vi "Dashboard Main.vi"() -> ()   [LabVIEW 2011]
uses:
  2013 Robot Code 11-1-12/Dashboard Datatype.ctl
  <vilib>/Rock Robotics/WPI/DriverStation/WPI_DriverStationDigitalData.ctl
panel:
  in  "Viewer":enum32{"Camera Image", "Kinect Skeleton", "IO"}(tab)
  in  "Video Left Enable":bool=TRUE
  out "Default Camera Left":T1(plugin-control)
  out "Camera Right":T1(plugin-control)
  in  "Video Right Enable":bool=TRUE
  out "Auton Name 1":string
  out "Auton Name 2":string
  out "Auton Name 3":string
  out "Auton Name 4":string
  out "Auton Name 5":string
  out "Auton Name 6":string
  out "Buttons 1":cluster{"1":bool, "2":bool, "3":bool}
  out "Kinect 1":cluster{"X":dbl, "Y":dbl, "Z":dbl} {"X" scale=1.0..-1.0; "Y" scale=1.0..-1.0; "Z" scale=1.0..-1.0}
  out "Buttons 2":cluster{"1":bool, "2":bool, "3":bool}
  out "Kinect 2":cluster{"X":dbl, "Y":dbl, "Z":dbl} {"X" scale=1.0..-1.0; "Y" scale=1.0..-1.0; "Z" scale=1.0..-1.0}
  out "Version":string
  out "Skeleton Picture":picture
  out "Players":i8
  out "PWM":cluster{u8, u8}[](array[slide])=[{0, 157}, {0, 157}, {0, 157}, {0, 157}, {0, 157}, {0, 157}, {0, 157}, {0, 157}, {0, 157}, {0, 169}] scale=1.0..255.0
  out "GPIO Output Enable":bool[](array[boolean])
  out "GPIO State":bool[](array[boolean])
  out "Relay":cluster{"Forward":bool[], "Reverse":bool[]}
  out "Solenoid Output":bool[](array[boolean])
  out "Robot IP Address":string
  out "8 -- Battery":sgl(graph)
  out "Analog Input":sgl[](array[slide]) scale=0.0..5.0
  out "Dashboard Datatype Warning":string="Warning: The Dashboard Datatype used by the robot project and this dashboard do not match.\nSee diagram for more details."
  out "Image Error Message":string="Timeout in Camera Communications"
  # "Digital #1"
  # "1"
  # "10"
  # "1"
  # "14"
  # "1"
  # "8"
  # "Solenoid #1"
  # "1"
  # "8"
  # "Communications"
  # "Analog #1"
  # "1"
  # "7"
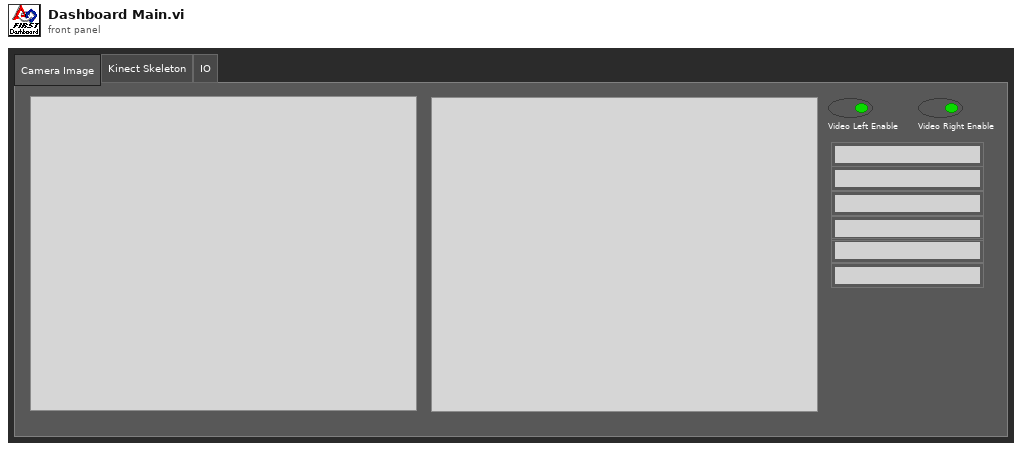
[diagram p1: front panel]
types:
  T1 = typedef "IMAQ Image.ctl" = refnum<image>
  T2 = typedef "Dashboard Datatype.ctl" = cluster{cluster{"AnalogModule[0]":cluster{"Channel[0]":sgl, "Channel[1]":sgl, "Channel[2]":sgl, "Channel[3]":sgl, "Channel[4]":sgl, "Channel[5]":sgl, "Channel[6]":sgl, "Channel[7]":sgl}, "AnalogModule[1]":cluster{"Channel[0]":sgl, "Channel[1]":sgl, "Channel[2]":sgl, "Channel[3]":sgl, "Channel[4]":sgl, "Channel[5]":sgl, "Channel[6]":sgl, "Channel[7]":sgl}}, cluster{"DigitalModule[0]":T3, "DigitalModule[1]":T3}, "Solenoid":u8, "Auton Files":string[]}
  T3 = typedef "WPI_DriverStationDigitalData.ctl" = cluster{"Relay Fwd":u8, "Relay Rev":u8, "GPIO":u16, "GPIO_OE":u16, "PWM":cluster{"PWM[0]":u8, "PWM[1]":u8, "PWM[2]":u8, "PWM[3]":u8, "PWM[4]":u8, "PWM[5]":u8, "PWM[6]":u8, "PWM[7]":u8, "PWM[8]":u8, "PWM[9]":u8}}
  T4 = typedef "Image Type" = u32
  T5 = cluster{"Competition mode":bool, "Robot Link":bool, "Autonomous":bool, "Enabled":bool, "E-Stop":bool}
  T6 = cluster{"AnalogModule[0]":cluster{"Channel[0]":sgl, "Channel[1]":sgl, "Channel[2]":sgl, "Channel[3]":sgl, "Channel[4]":sgl, "Channel[5]":sgl, "Channel[6]":sgl, "Channel[7]":sgl}, "AnalogModule[1]":cluster{"Channel[0]":sgl, "Channel[1]":sgl, "Channel[2]":sgl, "Channel[3]":sgl, "Channel[4]":sgl, "Channel[5]":sgl, "Channel[6]":sgl, "Channel[7]":sgl}}
  T7 = cluster{"DigitalModule[0]":T3, "DigitalModule[1]":T3}
  T8 = cluster{"Channel[0]":sgl, "Channel[1]":sgl, "Channel[2]":sgl, "Channel[3]":sgl, "Channel[4]":sgl, "Channel[5]":sgl, "Channel[6]":sgl, "Channel[7]":sgl}[]
  T9 = cluster{"Channel[0]":sgl, "Channel[1]":sgl, "Channel[2]":sgl, "Channel[3]":sgl, "Channel[4]":sgl, "Channel[5]":sgl, "Channel[6]":sgl, "Channel[7]":sgl}
  T10 = typedef "LVRectTypeDef.ctl" = cluster{"left":i16, "top":i16, "right":i16, "bottom":i16}
  T11 = typedef "SkeletonTrackState.ctl" = enum32{"NotTracked", "PositionOnly", "Tracked"}
  T12 = cluster{"TrackingState":u8[], "Position":cluster{"x":sgl, "y":sgl, "z":sgl}, cluster{"x":sgl, "y":sgl, "z":sgl, sgl}[], "TrackState":T11}
  T13 = cluster{cluster{"ScaledToPercentRange":dbl, "ScaledToPercentRange":dbl, "ScaledToPercentRange":dbl}, cluster{bool, bool, bool}}[]
  T14 = typedef "LVBoundsTypeDef.ctl" = cluster{"Width":u32, "Height":u32}
  T15 = cluster{cluster{"ScaledToPercentRange":dbl, "ScaledToPercentRange":dbl, "ScaledToPercentRange":dbl}, cluster{bool, bool, bool}}
  T16 = cluster{"ScaledToPercentRange":dbl, "ScaledToPercentRange":dbl, "ScaledToPercentRange":dbl}
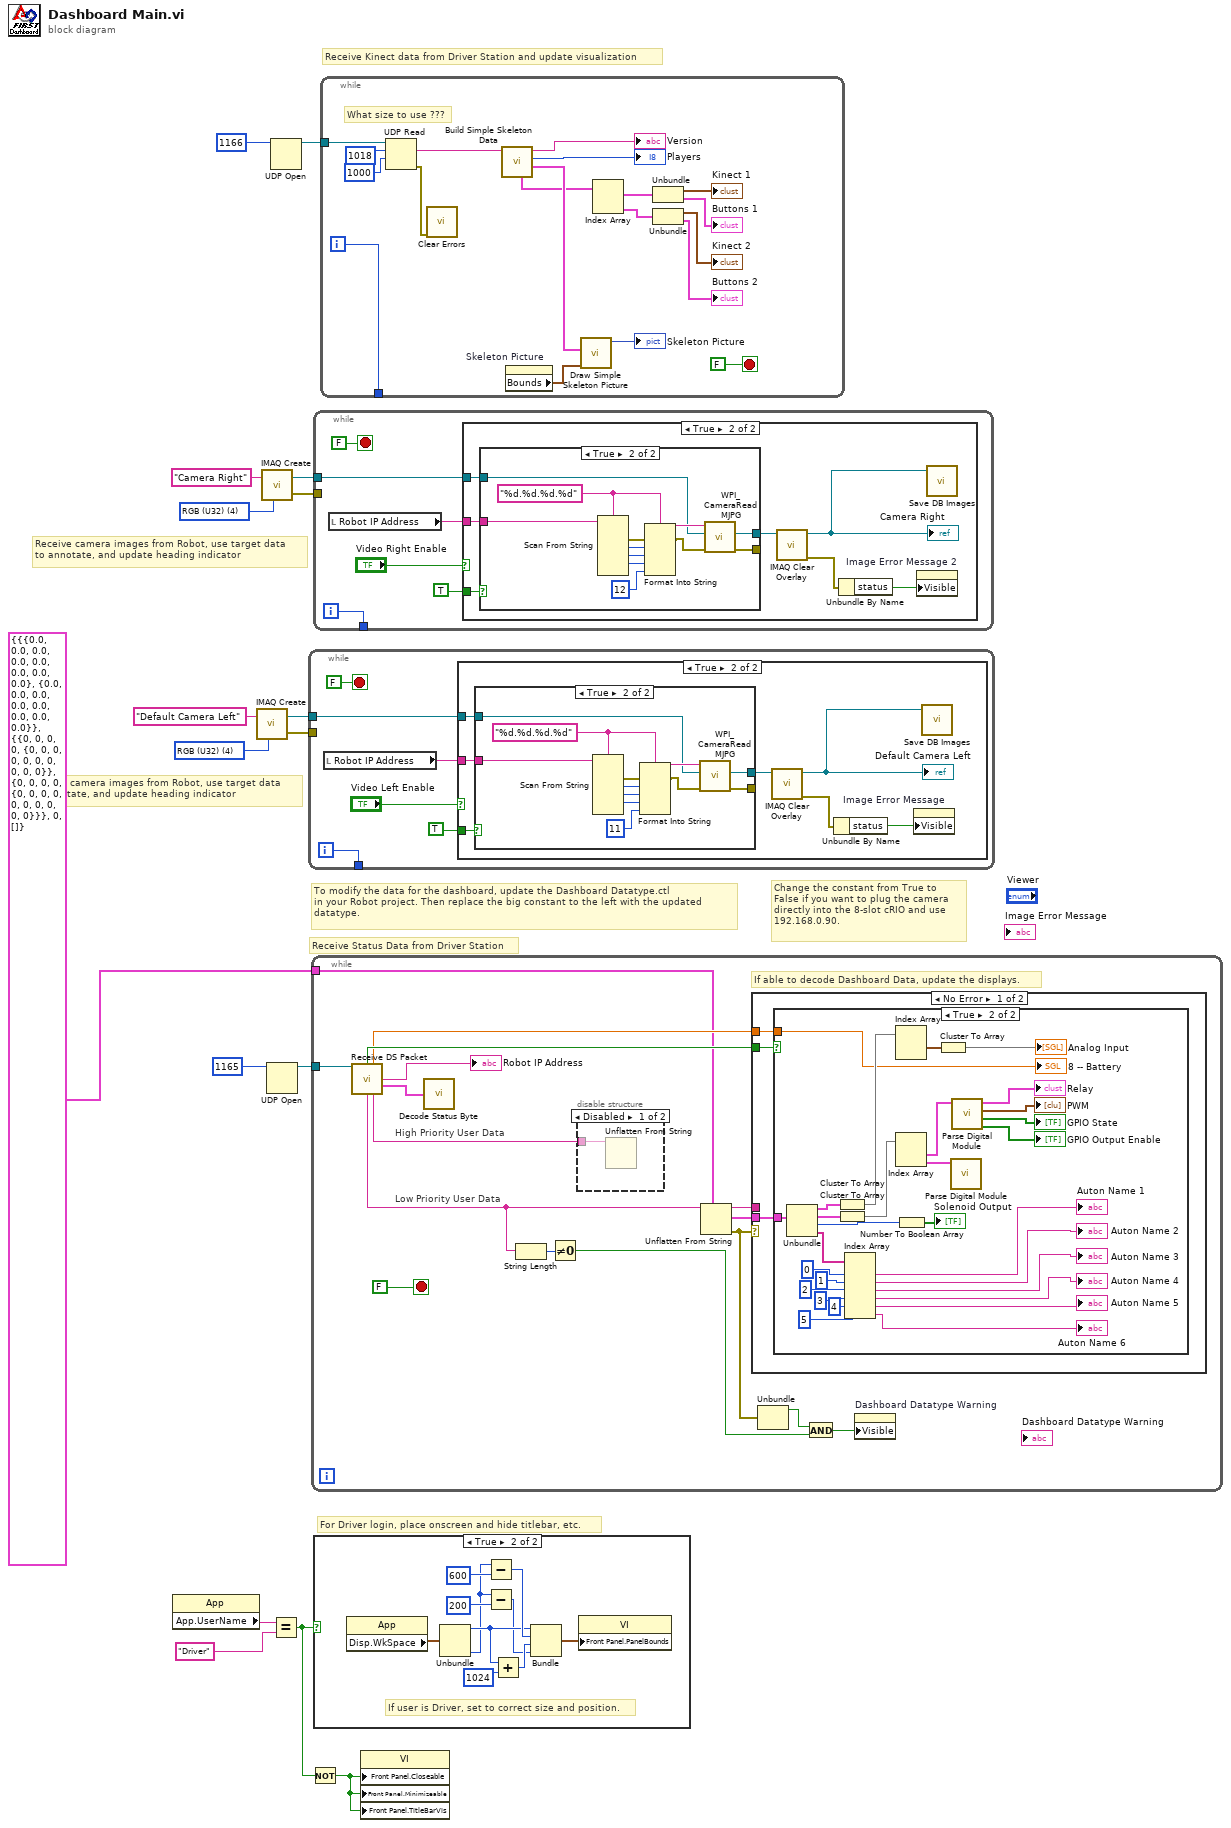
[diagram p0: block diagram]
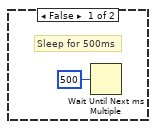
[diagram p2: hidden frame]
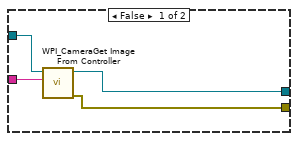
[diagram p3: hidden frame]
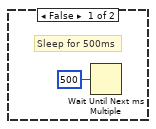
[diagram p8: hidden frame]
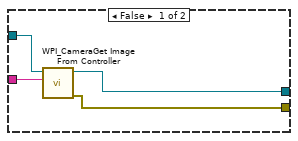
[diagram p9: hidden frame]
diagram:
  w5 = T4 4 items=["Grayscale (U8)", "Grayscale (I16)", "Grayscale (SGL)", "Complex (CSG)", "RGB (U32)", "HSL (U32)", "RGB (U64)"] ("Image Type")
  w15 = T4 4 items=["Grayscale (U8)", "Grayscale (I16)", "Grayscale (SGL)", "Complex (CSG)", "RGB (U32)", "HSL (U32)", "RGB (U64)"] ("Image Type")
  # "Receive camera images from Robot, use target data\nto annotate, and update heading indicator"
  # "Change the constant from True to\nFalse if you want to plug the camera\ndirectly into the 8-slot cRIO and use\n192.168.0.90."
  # "Receive Kinect data from Driver Station and update visualization"
  # "For Driver login, place onscreen and hide titlebar, etc."
  # "To modify the data for the dashboard, update the Dashboard Datatype.ctl\nin your Robot project. Then replace the big constant to the left with the updated\ndatatype."
  # "Receive Status Data from Driver Station"
  # "Receive camera images from Robot, use target data\nto annotate, and update heading indicator"
  n1 = property class="App"() -> ("App.UserName"=w10:string)  [unwired: 2 in, 2 out]
  n2 = call "IMAQ Create"("Image Name"="Default Camera Left", "Image Type"=w15) -> ("New Image"=w13:T1, "error out"=w12:errorcluster)  [unwired: 2 in, 1 out]
  n3 = call "IMAQ Create"("Image Name"="Camera Right", "Image Type"=w5) -> ("New Image"=w3:T1, "error out"=w2:errorcluster)  [unwired: 2 in, 1 out]
  n4 = UDP Open(11:u16 1165 ("port")) -> (port=w16:refnum<k16>)  [unwired: 2 in, 4 out]
  n5 = UDP Open(11:u16 1166 ("port")) -> (port=w6:refnum<k16>)  [unwired: 2 in, 4 out]
  n6 = Equal?(x=w10, y="Driver") -> (x = y?=w9:bool)
  n7 = while {
    tunnel: w13 -> [w21]
    tunnel: w12 -> [_]
    tunnel: [w18] -> _
    i -> [w18]
    stop <- FALSE stop-if-true
    n8 = local read "Robot IP Address"() -> (w22:string)
    n9 = case shown="True" "Video Left Enable" {
      tunnel: w22 -> [_ w31]
      tunnel: w21 -> [_ w30]
      tunnel: TRUE -> [_ w25]
      frame False {
        # "Sleep for 500ms"
        n10 = Wait Until Next ms Multiple(millisecond multiple=u32 500) -> ()  [unwired: 1 out]
      }
      frame True {
        n11 = case shown="True" w25 {
          tunnel: w30 -> [w34 w41]
          tunnel: [w32 w39] -> _
          tunnel: [w33 w40] -> w27
          tunnel: w31 -> [w35 w44]
          frame False {
            n12 = call <vilib>:"WPI_CameraGet Image From Controller.vi"("Controller Address"=w35, "Image"=w34) -> ("error out"=w32:errorcluster, "Image Out"=w33:T1)  [unwired: 2 in, 6 out]
          }
          frame True {
            w36 = "%d.%d.%d.%d" ("format string")
            n13 = Scan From String(format string=w36, input string=w44) -> (error out=w43:errorcluster, output 1=w45:i32, output 2=w46:i32, output 3=w47:i32)  [unwired: 2 in, 7 out]
            n14 = Format Into String(format string=w36, error in=w43, w45, w46, w47, 11 ("IP Suffix:")) -> (resulting string=w42:string, error out=w38:errorcluster)  [unwired: 1 in]
            n15 = call <vilib>:"WPI_CameraRead MJPG.vi"("error in"=w38, "Image"=w41, "address"=w42) -> ("error out"=w39:errorcluster, "Image Out"=w40:T1)  [unwired: 7 in]
          }
        }
        n16 = call "IMAQ Clear Overlay"("Image"=w27) -> ("error out"=w28:errorcluster, "Image Out"=w26:T1)  [unwired: 2 in, 7 out]
        "Default Camera Left" <- w26
        n17 = Unbundle By Name(w28) -> ("status"=w29:bool)
        n18 = property on="Image Error Message" class="Str"("Visible"=w29) -> ()  [unwired: 2 in, 2 out]
        n19 = call "Save DB Images.vi"("Image"=w26) -> ()  [unwired: 2 in, 1 out]
      }
    }
  }
  n20 = Not(x=w9) -> (.not. x?=w8:bool)
  n21 = while {
    tunnel: w16 -> [w61]
    tunnel: T2 {{"AnalogModule[0]"={"Channel[0]"=0.0, "Channel[1]"=0.0, "Channel[2]"=0.0, "Channel[3]"=0.0, "Channel[4]"=0.0, "Channel[5]"=0.0, "Channel[6]"=0.0, "Channel[7]"=0.0}, "AnalogModule[1]"={"Channel[0]"=0.0, "Channel[1]"=0.0, "Channel[2]"=0.0, "Channel[3]"=0.0, "Channel[4]"=0.0, "Channel[5]"=0.0, "Channel[6]"=0.0, "Channel[7]"=0.0}}, {"DigitalModule[0]"={"Relay Fwd"=0, "Relay Rev"=0, "GPIO"=0, "GPIO_OE"=0, "PWM"={"PWM[0]"=0, "PWM[1]"=0, "PWM[2]"=0, "PWM[3]"=0, "PWM[4]"=0, "PWM[5]"=0, "PWM[6]"=0, "PWM[7]"=0, "PWM[8]"=0, "PWM[9]"=0}}, "DigitalModule[1]"={"Relay Fwd"=0, "Relay Rev"=0, "GPIO"=0, "GPIO_OE"=0, "PWM"={"PWM[0]"=0, "PWM[1]"=0, "PWM[2]"=0, "PWM[3]"=0, "PWM[4]"=0, "PWM[5]"=0, "PWM[6]"=0, "PWM[7]"=0, "PWM[8]"=0, "PWM[9]"=0}}}, "Solenoid"=0, "Auton Files"=[]} ("Dashboard Data") -> [w48]
    stop <- FALSE stop-if-true
    # "High Priority User Data"
    # "Low Priority User Data"
    # "If able to decode Dashboard Data, update the displays."
    n22 = call "Receive DS Packet.vi"("Recv Socket"=w61) -> ("New Dashboard Data"=w58:bool, "Battery"=w49:sgl, "Robot IP Address"=→"Robot IP Address":string, "Status"=w62:T5, "Low Priority User Data"=w51:string, "High Priority User Data"=w50:string)  [unwired: 1 in, 8 out]
    n23 = call "Decode Status Byte.vi"("Status Byte"=w62) -> ()  [unwired: 2 out]
    n24 = String Length(string=w51) -> (length=w53:i32)
    n25 = Not Equal To 0?(x=w53) -> (x != 0?=w56:bool)
    n26 = disable-structure shown="Disabled" {
      disable-tunnel: w50 -> [w64 _]
      frame Disabled {
        n27 = Unflatten From String(binary string=w64) -> ()  [unwired: 2 in, 5 out]
      }
      frame Enabled {
      }
    }
    n28 = Unflatten From String(type=w48, binary string=w51) -> (rest of the binary string=w54:string, value=w60:T2, error out=w59:errorcluster)  [unwired: 1 in, 2 out]
    n29 = case shown="No Error" w59 {
      tunnel: w60 -> [w67 _]
      tunnel: w58 -> [w66 _]
      tunnel: w54 -> [_ _]
      tunnel: w49 -> [w65 _]
      frame No Error {
        n30 = case shown="True" w66 {
          tunnel: w67 -> [_ w87]
          tunnel: w65 -> [_ w81]
          frame False {
            # "Don't update if the robot hasn't sent new data"
          }
          frame True {
            n31 = Unbundle(w87) -> (w84:T6, w85:T7, "Solenoid"=w86:u8, "Auton Files"=w80:string[])
            n32 = Cluster To Array(cluster=w84) -> (array=w95:T8)
            n33 = Cluster To Array(cluster=w85) -> (array=w94:T3[])
            n34 = Index Array(array=w80, index #1=0 ("index"), index #2=1 ("index"), index #3=2 ("index"), index #4=3 ("index"), index #5=4 ("index"), index #6=5 ("index")) -> (element #1=→"Auton Name 1":string, element #2=→"Auton Name 2":string, element #3=→"Auton Name 3":string, element #4=→"Auton Name 4":string, element #5=→"Auton Name 5":string, element #6=→"Auton Name 6":string)
            n35 = Index Array(array=w95) -> (element #1=w82:T9)  [unwired: 2 in, 1 out]
            n36 = Index Array(array=w94) -> (element #1=w93:T3, element #2=w88:T3)  [unwired: 2 in]
            n37 = Number To Boolean Array(number=w86) -> (Boolean array=→"Solenoid Output":bool[])
            n38 = Cluster To Array(cluster=w82) -> (array=→"Analog Input":sgl[])
            n39 = call "Parse Digital Module.vi"("DigitalModule"=w88) -> ()  [unwired: 11 out]
            n40 = call "Parse Digital Module.vi"("DigitalModule"=w93) -> ("GPIO Output Enable"=→"GPIO Output Enable":bool[], "GPIO State"=→"GPIO State":bool[], "PWM"=→"PWM":cluster{u8, u8}[], "Relay"=→"Relay":cluster{"Forward":bool[], "Reverse":bool[]})  [unwired: 7 out]
            "8 -- Battery" <- w81
          }
        }
      }
      frame Error {
        # "Your datatypes don't match. The Dashboard Datatype.ctl in your Robot project\nand the big constant to the left of the loop need to match."
      }
    }
    n41 = Unbundle(w59) -> ("status"=w55:bool)  [unwired: 2 out]
    n42 = And(x=w55, y=w56) -> (x .and. y?=w57:bool)
    n43 = property on="Dashboard Datatype Warning" class="Str"("Visible"=w57) -> ()  [unwired: 2 in, 2 out]
  }
  n44 = while {
    tunnel: w3 -> [w100]
    tunnel: w2 -> [_]
    tunnel: [w97] -> _
    i -> [w97]
    stop <- FALSE stop-if-true
    n45 = local read "Robot IP Address"() -> (w101:string)
    n46 = case shown="True" "Video Right Enable" {
      tunnel: w101 -> [_ w110]
      tunnel: w100 -> [_ w109]
      tunnel: TRUE -> [_ w105]
      frame False {
        # "Sleep for 500ms"
        n47 = Wait Until Next ms Multiple(millisecond multiple=u32 500) -> ()  [unwired: 1 out]
      }
      frame True {
        n48 = case shown="True" w105 {
          tunnel: w109 -> [w113 w120]
          tunnel: [w111 w118] -> _
          tunnel: [w112 w119] -> w107
          tunnel: w110 -> [w114 w123]
          frame False {
            n49 = call <vilib>:"WPI_CameraGet Image From Controller.vi"("Controller Address"=w114, "Image"=w113) -> ("error out"=w111:errorcluster, "Image Out"=w112:T1)  [unwired: 2 in, 6 out]
          }
          frame True {
            w115 = "%d.%d.%d.%d" ("format string")
            n50 = Scan From String(format string=w115, input string=w123) -> (error out=w122:errorcluster, output 1=w124:i32, output 2=w125:i32, output 3=w126:i32)  [unwired: 2 in, 7 out]
            n51 = Format Into String(format string=w115, error in=w122, w124, w125, w126, 12 ("IP Suffix:")) -> (resulting string=w121:string, error out=w117:errorcluster)  [unwired: 1 in]
            n52 = call <vilib>:"WPI_CameraRead MJPG.vi"("error in"=w117, "Image"=w120, "address"=w121) -> ("error out"=w118:errorcluster, "Image Out"=w119:T1)  [unwired: 7 in]
          }
        }
        n53 = call "IMAQ Clear Overlay"("Image"=w107) -> ("error out"=w108:errorcluster, "Image Out"=w106:T1)  [unwired: 2 in, 7 out]
        "Camera Right" <- w106
        n54 = Unbundle By Name(w108) -> ("status"=w104:bool)
        n55 = property on="Image Error Message 2" class="Str"("Visible"=w104) -> ()  [unwired: 2 in, 2 out]
        n56 = call "Save DB Images.vi"("Image"=w106) -> ()  [unwired: 2 in, 1 out]
      }
    }
  }
  n57 = case shown="True" w9 {
    frame False {
    }
    frame True {
      # "If user is Driver, set to correct size and position."
      n58 = property class="App"() -> ("Disp.WkSpace"=w136:T10)  [unwired: 2 in, 2 out]
      n59 = Unbundle(w136) -> ("left"=w131:i16, "bottom"=w127:i16)  [unwired: 2 out]
      n60 = Subtract(x=w127, y=600) -> (x-y=w133:i32)
      n61 = Subtract(x=w127, y=200) -> (x-y=w128:i32)
      n62 = Add(x=w131, y=1024) -> (x+y=w132:i32)
      n63 = Bundle("left"=w131, w133, w132, w128) -> (w135:cluster{"left":i16, i32, i32, i32})  [unwired: 1 out]
      n64 = property class="VI"("Front Panel.PanelBounds"=w135) -> ()  [unwired: 2 in, 2 out]
    }
  }
  n65 = while {
    tunnel: w6 -> [w153]
    tunnel: [w137] -> _
    i -> [w137]
    stop <- FALSE stop-if-true
    # "What size to use ???"
    n66 = UDP Read(connection ID=w153, max size (548)=1018 ("bytes to read"), timeout ms (25000)=1000) -> (data out=w147:string, error out=w145:errorcluster)  [unwired: 1 in, 3 out]
    n67 = call <vilib>:"Clear Errors.vi"("error in (no error)"=w145) -> ()  [unwired: 6 in, 1 out]
    n68 = call "Build Simple Skeleton Data.vi"("data out"=w147) -> ("Skeleton Data"=w148:T12, "NumPlayers"=→"Players":i8, "Version String"=→"Version":string, "Simple Joystick Info"=w144:T13)  [unwired: 6 in, 1 out]
    n69 = property on="Skeleton Picture" class="Pict"() -> ("Bounds"=w149:T14)  [unwired: 2 in, 2 out]
    n70 = call "Draw Simple Skeleton Picture.vi"("Bounds"=w149, "Simple Skeleton"=w148) -> ("new picture out"=→"Skeleton Picture":picture)  [unwired: 9 in]
    n71 = Index Array(array=w144) -> (element #1=w143:T15, element #2=w142:T15)  [unwired: 2 in]
    n72 = Unbundle(w143) -> (→"Kinect 1":T16, →"Buttons 1":cluster{bool, bool, bool})
    n73 = Unbundle(w142) -> (→"Kinect 2":T16, →"Buttons 2":cluster{bool, bool, bool})
  }
  n74 = property class="VI"("Front Panel.Closeable"=w8, "Front Panel.Minimizeable"=w8, "Front Panel.TitleBarVis"=w8) -> ()  [unwired: 2 in, 2 out]
